vi "流量计通讯.vi"() -> ()   [LabVIEW 2016, in "流量计集成.lvlib" / "WL1A1明渠流量计.lvlib"]
uses:
  <vilib>/Platform/TimedLoop/XDataNode/timing_clust.ctl
  <vilib>/Platform/TimedLoop/XDataNode/nitl_modes.ctl
  <vilib>/Platform/TimedLoop/XDataNode/wakeup.ctl
  <vilib>/Plasmionique/MB Master/MB_ADU/MB_ADU.lvclass/MB_ADU.ctl
  <vilib>/Plasmionique/MB Master/MB_ADU/Read TX Timestamp.vi
  <vilib>/Plasmionique/MB Master/MB_ADU/Read TX Data.vi
  <vilib>/Plasmionique/MB Master/MB_ADU/Read RX Timestamp.vi
  <vilib>/Plasmionique/MB Master/MB_ADU/Read RX Data.vi
  <vilib>/Plasmionique/MB Master/MB_Master_Serial/MB_Master_Serial.lvclass
  D:/Program Files (x86)/National Instruments/LabVIEW 2016/vi.lib/Plasmionique/MB Master/MB_Master/MB_Master.lvclass
  <vilib>/Platform/TimedLoop/XDataNode/XDataNode.xnode
  <vilib>/Plasmionique/MB Master/MB_ADU/MB_ADU.lvclass
  <vilib>/Platform/TimedLoop/XDataNode/XDNodeRunTimeDep.lvlib
  <vilib>/Plasmionique/MB Master/MB Master.lvlib
panel:
  out "RX":string
  out "TX":string
  in  "停止":bool
  out "显示值":T1
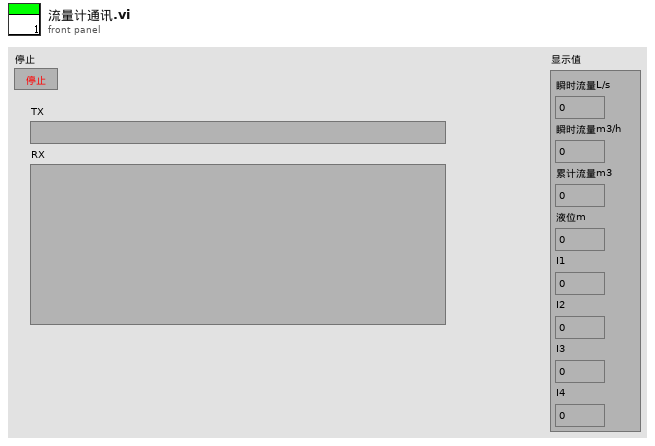
[diagram p1: front panel]
types:
  T1 = cluster{"瞬时流量L/s":dbl, "瞬时流量m3/h":dbl, "累计流量m3":dbl, "液位m":dbl, "I1":dbl, "I2":dbl, "I3":dbl, "I4":dbl}
  T2 = cluster{"baud rate (bps)":u32, "stop bits":u16, "parity":u16, "flow control":u16, "timeout":u32, "retries":i32}
  T3 = typedef "XDNodeRunTimeDep.lvlib/timing_clust.ctl" = cluster{"Expected End [f-1]":u64, "Actual End [f-1]":u64, "Finished Late? [f-1]":bool, "Expected End [i-1]":u64, "Actual End [i-1]":u64, "Finished Late? [i-1]":bool, "Expected Start [i]":u64, "Actual Start [i]":u64, "Expected Start [f]":u64, "Actual Start [f]":u64, "Source Name":string, "Structure Name":string, "Period":i64, "Deadline":i64, "Offset":i64, "Start":i64, "Priority":i32, "Timeout":i32, "Mode":T4, "Wakeup Reason":T5, "Error":errorcluster, "Source Type":string, "Secondary Source Type":string, "Global End Time":u64, "Global Start Time":u64, "Frame Duration":u64, "Iteration Duration":u64, "Assigned CPU":i32, "I/O Scan Engine Mode":u32}
  T4 = typedef "XDNodeRunTimeDep.lvlib/nitl_modes.ctl" = enum32{"No Change", "Process missed periods, maintain original phase", "Discard missed periods, maintain original phase", "Process missed periods, ignore original phase", "Discard missed periods, ignore original phase"}
  T5 = typedef "XDNodeRunTimeDep.lvlib/wakeup.ctl" = enum32{"Normal", "Aborted", "Asynchronous wakeup", "Timing source error", "Timed loop error", "Timeout"}
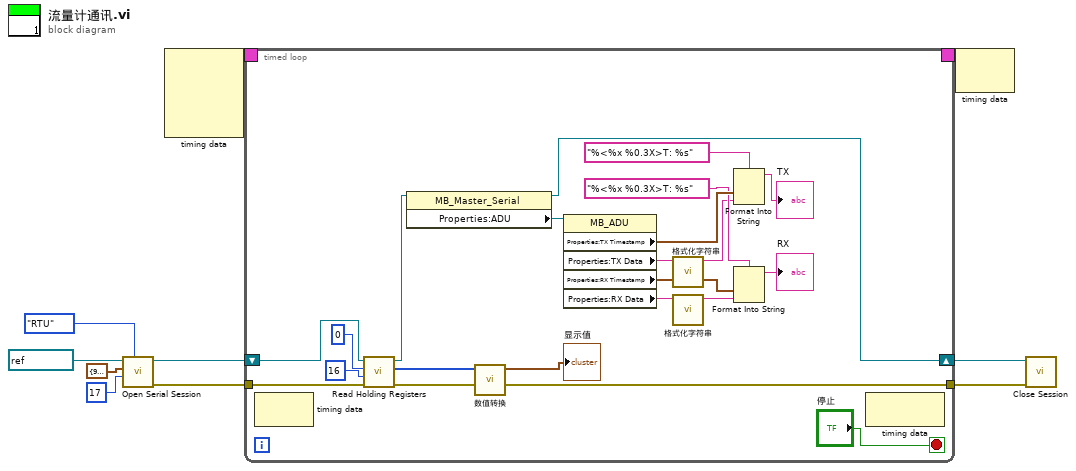
[diagram p0: block diagram]
diagram:
  n1 = call <vilib>:"Open Serial Session.vi"("Mode (RTU)"=enum16{"RTU", "ASCII"}."RTU", "Slave ID"=u8 17, "Serial Config"=T2 {"baud rate (bps)"=9600, "stop bits"=10, "parity"=2, "flow control"=0, "timeout"=1000, "retries"=1}, "VISA Resource"=refnum<visa-resource-name> "COM7") -> ("Error out"=w5:errorcluster, "MB_Serial session"=w6:refnum<class "MB_Master_Serial.lvclass">)  [unwired: 6 in]
  n2 = node-c288() -> (w10:T3)  [unwired: 4 in]
  n3 = timed-loop {
    timing: w10 -> [_]
    timing-out: [_] -> w9
    tunnel: w5 -> [w31]
    shift-right: [w22] -> w8
    shift-left: w6 -> [w25]
    tunnel: [w28] -> w7
    stop <- "停止" stop-if-true
    n4 = node-c288() -> ()  [unwired: 1 in, 1 out]
    n5 = call <vilib>:"Read Holding Registers.vi"("error in (no error)"=w31, "quantity"=u16 16, "starting address"=u16 0, "MB session in"=w25) -> ("error out"=w28:errorcluster, "Registers"=w27:u16[], "MB session out"=w23:refnum<class "MB_Master_Serial.lvclass">)  [unwired: 5 in]
    n6 = property class="MB_Master_Serial"(reference=w23) -> (reference out=w22:refnum<class "MB_Master_Serial.lvclass">, "Properties:ADU"=w21:refnum<class "MB_ADU.lvclass">)  [unwired: 1 in, 1 out]
    n7 = call "数值转换.vi"("数组"=w27) -> ("显示值"=→"显示值":T1)  [unwired: 10 in]
    n8 = property class="MB_ADU"(reference=w21) -> ("Properties:TX Timestamp"=w19:timestamp, "Properties:TX Data"=w14:string, "Properties:RX Timestamp"=w17:timestamp, "Properties:RX Data"=w12:string)  [unwired: 1 in, 2 out]
    n9 = call "格式化字符串.vi"("字符串"=w14) -> ("字符串 2"=w13:string)  [unwired: 10 in]
    n10 = call "格式化字符串.vi"("字符串"=w12) -> ("字符串 2"=w11:string)  [unwired: 10 in]
    n11 = Format Into String(format string="%<%x %0.3X>T: %s" ("格式字符串"), w19, w13) -> (resulting string=→"TX":string)  [unwired: 2 in, 1 out]
    n12 = Format Into String(format string="%<%x %0.3X>T: %s" ("格式字符串"), w17, w11) -> (resulting string=→"RX":string)  [unwired: 2 in, 1 out]
    n13 = node-c288() -> ()  [unwired: 1 in, 1 out]
  }
  n14 = node-c288(w9) -> ()  [unwired: 1 out]
  n15 = call-dynamic "Close Session.vi"("error in (no error)"=w7, "MB_Serial session"=w8) -> ()  [unwired: 9 in, 1 out]
